vi "GetWavelength.vi"(8 "error in (no error)":errorcluster, 11 "Device Index":u8) -> (0 "error out":errorcluster, 1 "Wavelength Code":u8, 2 "Wavelength":dbl, 3 "Device Index":u8)   [LabVIEW 2019, in "TopasDriver.lvlib"]
uses:
  TopasDriver.lvlib
  TopasAPI.dll
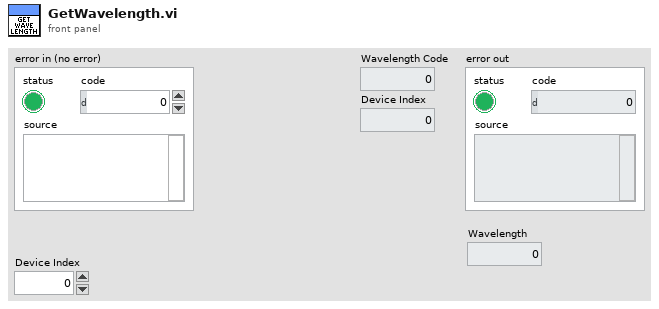
[diagram p1: front panel]
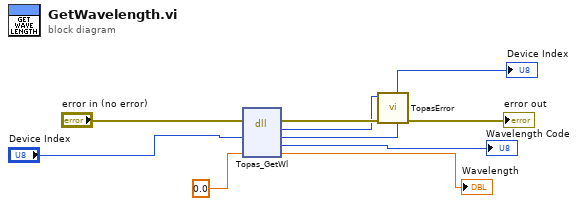
[diagram p0: block diagram]
diagram:
  n1 = dll-call lib="G:/LabVIEW/Topas-LabVIEW-Driver/Libraries/TopasAPI.dll" fn="Topas_GetWl"(error in="error in (no error)", "index"="Device Index", "wl"=0.0) -> (error out=w7:errorcluster, "return type"=w5:u32, "index"=→"Device Index":u8, "wl_code"=→"Wavelength Code":u8, "wl"=→"Wavelength":dbl)  [unwired: 3 in, 1 out]
  n2 = call "TopasError.vi"("error in"=w7, "Error Code"=w5) -> ("error out"=→"error out":errorcluster)  [unwired: 9 in]
